vi "p1.vi"() -> ()   [LabVIEW 2021, in "d22.lvlib"]
uses:
  d22.lvlib
  AOC/AOC.lvlib
panel:
  out "facing":enum16{"R", "D", "L", "U"}(ring)=enum."L"
  out "col":i32=43
  out "row":i32=133
  in  "Example":string="        ...#\n        .#..\n        #...\n        ....\n...#.......#\n........#...\n..#....#....\n..........#.\n        ...#....\n        .....#..\n        .#......\n        ......#.\n\n10R5L5R10L4R5L5"
  in  "Example":bool
  out "Answer":i64=133174
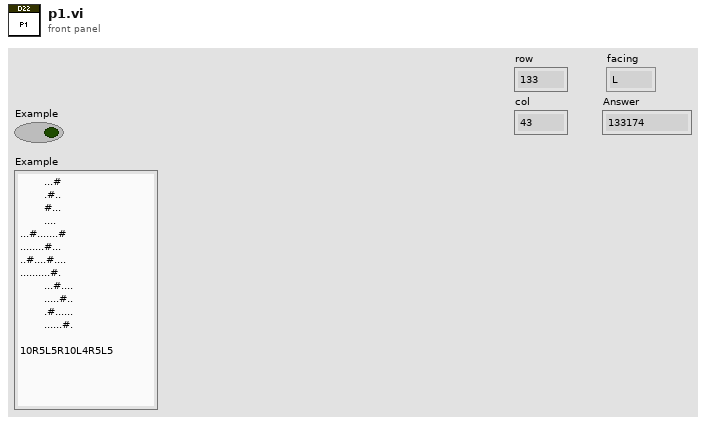
[diagram p1: front panel]
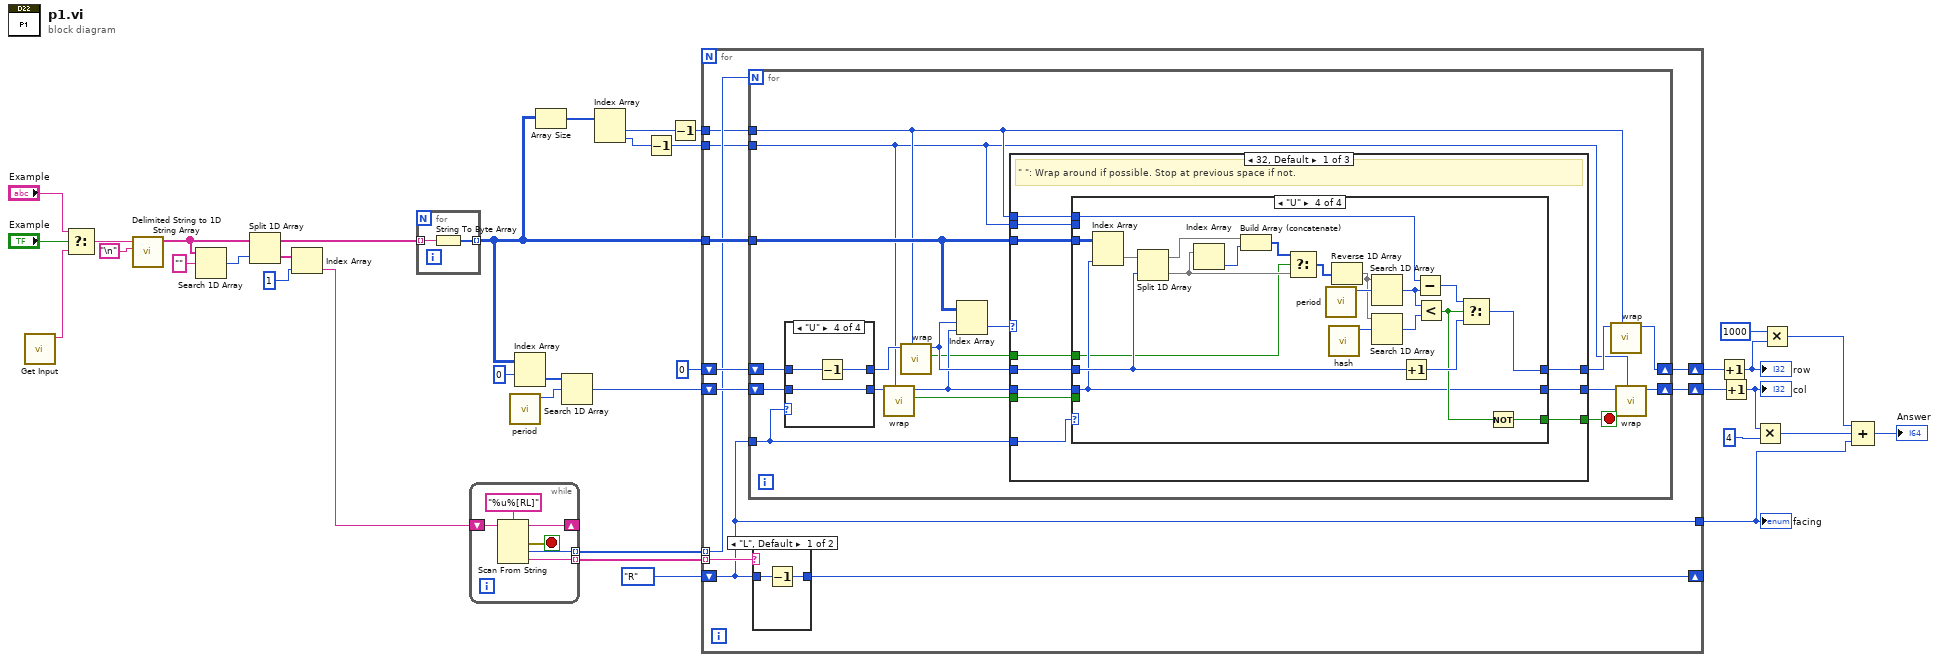
[diagram p0: block diagram]
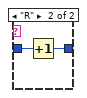
[diagram p2: hidden frame]
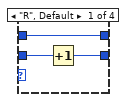
[diagram p3: hidden frame]
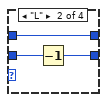
[diagram p4: hidden frame]
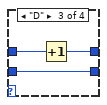
[diagram p5: hidden frame]
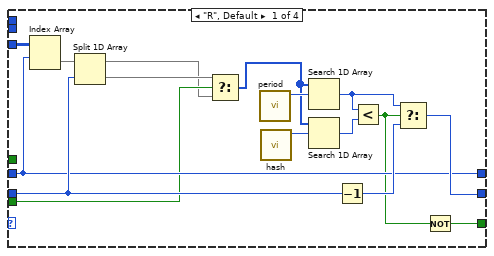
[diagram p6: hidden frame]
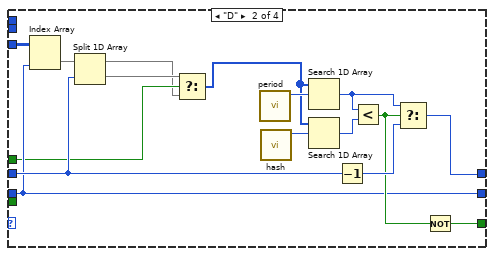
[diagram p7: hidden frame]
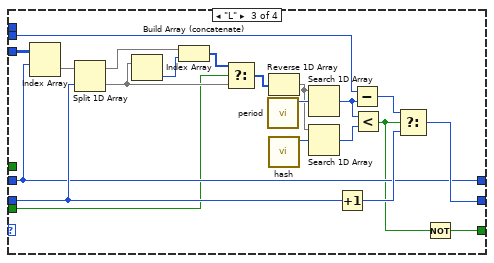
[diagram p8: hidden frame]
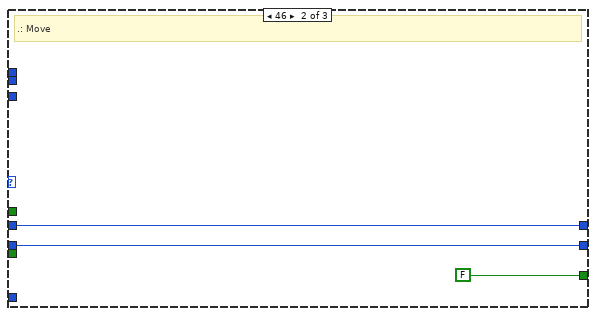
[diagram p9: hidden frame]
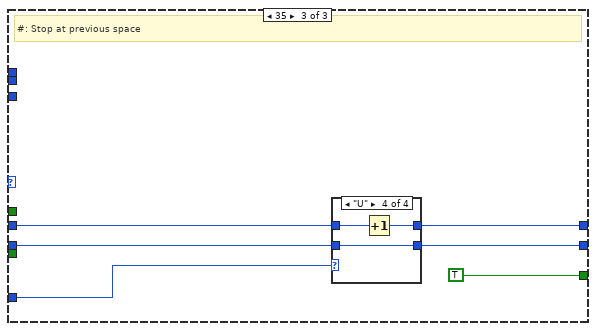
[diagram p10: hidden frame]
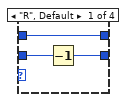
[diagram p11: hidden frame]
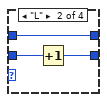
[diagram p12: hidden frame]
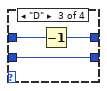
[diagram p13: hidden frame]
diagram:
  n1 = call "Get Input.vi"() -> ("Input"=w36:string)  [unwired: 11 in]
  n2 = Select(t="Example", s="Example", f=w36) -> (s? t:f=w35:string)
  n3 = call <vilib>:"Delimited String to 1D String Array.vi"("delimiter"="\n", "delimited string"=w35) -> ("string array"=w28:string[])  [unwired: 9 in]
  n4 = Search 1D Array(1D array=w28, element="") -> (index of element=w26:i32)  [unwired: 1 in]
  n5 = Split 1D Array(array=w28, index=w26) -> (first subarray=w27:string[], second subarray=w23:string[])
  n6 = Index Array(array=w23, index=1) -> (element=w21:string)
  n7 = for {
    tunnel: w27 -> [w38] mode=indexing
    tunnel: [w37] -> w16 mode=indexing
    n8 = String To Byte Array(string=w38) -> (unsigned byte array=w37:u8[])
  }
  n9 = while {
    shift-right: [w39] -> _
    shift-left: w21 -> [w44]
    tunnel: [w41] -> w19 mode=indexing
    tunnel: [w42] -> w20 mode=indexing
    stop <- w40 stop-if-true
    n10 = Scan From String(format string="%u%[RL]", input string=w44) -> (remaining string=w39:string, error out=w40:errorcluster, output 1=w42:u32, output 2=w41:string)  [unwired: 4 in, 1 out]
  }
  n11 = call "period.vi"() -> ("."=w17:u8)  [unwired: 11 in]
  n12 = Index Array(array=w16, index (row)=0) -> (element=w30:u8[])  [unwired: 1 in]
  n13 = Array Size(array=w16) -> (size(s)=w15:i32[])
  n14 = Search 1D Array(1D array=w30, element=w17) -> (index of element=w25:i32)  [unwired: 1 in]
  n15 = Index Array(array=w15) -> (element #1=w4:i32, element #2=w2:i32)  [unwired: 2 in]
  n16 = Decrement(x=w2) -> (x-1=w1:i32)
  n17 = Decrement(x=w4) -> (x-1=w3:i32)
  n18 = for {
    tunnel: w16 -> [w52]
    shift-right: [w48] -> w13
    shift-left: w25 -> [w54]
    shift-right: [w49] -> w14
    shift-left: 0 ("index of element") -> [w55]
    tunnel: w20 -> [w51] mode=indexing
    tunnel: w19 -> [w50] mode=indexing
    shift-right: [w53] -> _
    shift-left: enum16{"R", "D", "L", "U"}."R" -> [w47]
    tunnel: [w47] -> w6
    tunnel: w3 -> [w46]
    tunnel: w1 -> [w45]
    n19 = for {
      N: w51 -> [_]
      tunnel: w47 -> [w73]
      tunnel: w52 -> [w72]
      shift-right: [w64] -> w48
      shift-left: w54 -> [w77]
      shift-right: [w66] -> w49
      shift-left: w55 -> [w76]
      tunnel: w46 -> [w61]
      tunnel: w45 -> [w60]
      stop <- w74 stop-if-true
      n20 = case shown="\"U\"" w73 {
        tunnel: w77 -> [w79 w82 w86 w89]
        tunnel: w76 -> [w80 w83 w85 w88]
        tunnel: [w80 w83 w84 w87] -> w71
        tunnel: [w78 w81 w86 w89] -> w69
        frame "R", Default {
          n21 = Increment(x=w79) -> (x+1=w78:i32)
        }
        frame "L" {
          n22 = Decrement(x=w82) -> (x-1=w81:i32)
        }
        frame "D" {
          n23 = Increment(x=w85) -> (x+1=w84:i32)
        }
        frame "U" {
          n24 = Decrement(x=w88) -> (x-1=w87:i32)
        }
      }
      n25 = call "wrap.vi"("Max"=w60, "value"=w69) -> ("wrapped?"=w62:bool, "wrapped value"=w68:i32)  [unwired: 8 in]
      n26 = call "wrap.vi"("Max"=w61, "value"=w71) -> ("wrapped?"=w63:bool, "wrapped value"=w70:i32)  [unwired: 8 in]
      n27 = Index Array(array=w72, index (row)=w70, index (col)=w68) -> (element=w75:u8)
      n28 = case shown="32, Default" w75 {
        tunnel: w70 -> [w99 w176 w182]
        tunnel: w68 -> [w97 w177 w180]
        tunnel: [w98 w177 w179] -> w65
        tunnel: [w95 w176 w181] -> w67
        tunnel: [w94 FALSE TRUE] -> w74
        tunnel: w73 -> [w96 _ w178]
        tunnel: w72 -> [w100 _ _]
        tunnel: w61 -> [w93 _ _]
        tunnel: w60 -> [w92 _ _]
        tunnel: w63 -> [w91 _ _]
        tunnel: w62 -> [w90 _ _]
        frame 32, Default {
          # "\" \": Wrap around if possible. Stop at previous space if not."
          n29 = case shown="\"U\"" w96 {
            tunnel: w100 -> [w116 w132 w153 w174]
            tunnel: w99 -> [w107 w123 w144 w163]
            tunnel: [w110 w121 w147 w161] -> w98
            tunnel: w97 -> [w109 w121 w146 w161]
            tunnel: [w107 w122 w144 w162] -> w95
            tunnel: [w105 w124 w142 w166] -> w94
            tunnel: w93 -> [_ _ _ w154]
            tunnel: w92 -> [_ _ w133 _]
            tunnel: w91 -> [_ w120 _ w155]
            tunnel: w90 -> [w103 _ w134 _]
            frame "R", Default {
              n30 = Index Array(array=w116, index (row)=w107) -> (element=w115:u8[])  [unwired: 1 in]
              n31 = Split 1D Array(array=w115, index=w109) -> (first subarray=w102:u8[], second subarray=w104:u8[])
              n32 = Select(t=w104, s=w103, f=w102) -> (s? t:f=w101:u8[])
              n33 = call "period.vi"() -> ("."=w114:u8)  [unwired: 11 in]
              n34 = call "hash.vi"() -> ("#"=w113:u8)  [unwired: 11 in]
              n35 = Search 1D Array(1D array=w101, element=w114) -> (index of element=w111:i32)  [unwired: 1 in]
              n36 = Search 1D Array(1D array=w101, element=w113) -> (index of element=w112:i32)  [unwired: 1 in]
              n37 = Decrement(x=w109) -> (x-1=w108:i32)
              n38 = Less?(x=w111, y=w112) -> (x < y?=w106:bool)
              n39 = Select(t=w111, s=w106, f=w108) -> (s? t:f=w110:i32)
              n40 = Not(x=w106) -> (.not. x?=w105:bool)
            }
            frame "D" {
              n41 = Index Array(array=w132, index (col)=w121) -> (element=w131:u8[])  [unwired: 1 in]
              n42 = Split 1D Array(array=w131, index=w123) -> (first subarray=w118:u8[], second subarray=w119:u8[])
              n43 = Select(t=w119, s=w120, f=w118) -> (s? t:f=w117:u8[])
              n44 = call "period.vi"() -> ("."=w130:u8)  [unwired: 11 in]
              n45 = call "hash.vi"() -> ("#"=w129:u8)  [unwired: 11 in]
              n46 = Search 1D Array(1D array=w117, element=w130) -> (index of element=w127:i32)  [unwired: 1 in]
              n47 = Search 1D Array(1D array=w117, element=w129) -> (index of element=w128:i32)  [unwired: 1 in]
              n48 = Decrement(x=w123) -> (x-1=w126:i32)
              n49 = Less?(x=w127, y=w128) -> (x < y?=w125:bool)
              n50 = Select(t=w127, s=w125, f=w126) -> (s? t:f=w122:i32)
              n51 = Not(x=w125) -> (.not. x?=w124:bool)
            }
            frame "L" {
              n52 = Index Array(array=w153, index (row)=w144) -> (element=w152:u8[])  [unwired: 1 in]
              n53 = Split 1D Array(array=w152, index=w146) -> (first subarray=w137:u8[], second subarray=w136:u8[])
              n54 = Index Array(array=w136) -> (element=w138:u8)  [unwired: 1 in]
              n55 = Build Array (concatenate)(w137, w138) -> (w139:u8[])
              n56 = Select(t=w139, s=w134, f=w136) -> (s? t:f=w135:u8[])
              n57 = call "period.vi"() -> ("."=w151:u8)  [unwired: 11 in]
              n58 = Reverse 1D Array(array=w135) -> (reversed array=w141:u8[])
              n59 = call "hash.vi"() -> ("#"=w150:u8)  [unwired: 11 in]
              n60 = Search 1D Array(1D array=w141, element=w151) -> (index of element=w148:i32)  [unwired: 1 in]
              n61 = Search 1D Array(1D array=w141, element=w150) -> (index of element=w149:i32)  [unwired: 1 in]
              n62 = Increment(x=w146) -> (x+1=w145:i32)
              n63 = Subtract(x=w133, y=w148) -> (x-y=w140:i32)
              n64 = Less?(x=w148, y=w149) -> (x < y?=w143:bool)
              n65 = Select(t=w140, s=w143, f=w145) -> (s? t:f=w147:i32)
              n66 = Not(x=w143) -> (.not. x?=w142:bool)
            }
            frame "U" {
              n67 = Index Array(array=w174, index (col)=w161) -> (element=w173:u8[])  [unwired: 1 in]
              n68 = Split 1D Array(array=w173, index=w163) -> (first subarray=w160:u8[], second subarray=w157:u8[])
              n69 = Index Array(array=w157) -> (element=w156:u8)  [unwired: 1 in]
              n70 = Build Array (concatenate)(w160, w156) -> (w158:u8[])
              n71 = Select(t=w158, s=w155, f=w157) -> (s? t:f=w159:u8[])
              n72 = call "period.vi"() -> ("."=w172:u8)  [unwired: 11 in]
              n73 = call "hash.vi"() -> ("#"=w171:u8)  [unwired: 11 in]
              n74 = Reverse 1D Array(array=w159) -> (reversed array=w165:u8[])
              n75 = Search 1D Array(1D array=w165, element=w172) -> (index of element=w169:i32)  [unwired: 1 in]
              n76 = Search 1D Array(1D array=w165, element=w171) -> (index of element=w170:i32)  [unwired: 1 in]
              n77 = Increment(x=w163) -> (x+1=w168:i32)
              n78 = Subtract(x=w154, y=w169) -> (x-y=w164:i32)
              n79 = Less?(x=w169, y=w170) -> (x < y?=w167:bool)
              n80 = Select(t=w164, s=w167, f=w168) -> (s? t:f=w162:i32)
              n81 = Not(x=w167) -> (.not. x?=w166:bool)
            }
          }
        }
        frame 46 {
          # ".: Move"
        }
        frame 35 {
          # "#: Stop at previous space"
          n82 = case shown="\"U\"" w178 {
            tunnel: w180 -> [w185 w188 w192 w195]
            tunnel: w182 -> [w186 w189 w191 w194]
            tunnel: [w186 w189 w190 w193] -> w181
            tunnel: [w184 w187 w192 w195] -> w179
            frame "R", Default {
              n83 = Decrement(x=w185) -> (x-1=w184:i32)
            }
            frame "L" {
              n84 = Increment(x=w188) -> (x+1=w187:i32)
            }
            frame "D" {
              n85 = Decrement(x=w191) -> (x-1=w190:i32)
            }
            frame "U" {
              n86 = Increment(x=w194) -> (x+1=w193:i32)
            }
          }
        }
      }
      n87 = call "wrap.vi"("Max"=w61, "value"=w67) -> ("wrapped value"=w66:i32)  [unwired: 8 in, 1 out]
      n88 = call "wrap.vi"("Max"=w60, "value"=w65) -> ("wrapped value"=w64:i32)  [unwired: 8 in, 1 out]
    }
    n89 = case shown="\"L\", Default" w50 {
      tunnel: [w56 w59] -> w53
      tunnel: w47 -> [w57 w58]
      frame "L", Default {
        n90 = Decrement(x=w57) -> (x-1=w56:enum16{"R", "D", "L", "U"})
      }
      frame "R" {
        n91 = Increment(x=w58) -> (x+1=w59:enum16{"R", "D", "L", "U"})
      }
    }
  }
  "facing" <- w6
  n92 = Increment(x=w14) -> (x+1=w12:i32)
  "row" <- w12
  n93 = Increment(x=w13) -> (x+1=w10:i32)
  "col" <- w10
  n94 = Multiply(x=w10, y=4 ("x+1")) -> (x*y=w7:i32)
  n95 = Multiply(x=1000, y=w12) -> (x*y=w8:i32)
  n96 = Compound Arithmetic op=ADD(w8, w7, w6) -> (→"Answer":i32)
